vi "Create Hyperlink between 2 sheets.vi"(0 "Work Sheet":refnum<k7>, 1 "Sheet Name 2":string, 2 "Sheet Name 1":string, 3 "Link Cell 1":string, 4 "Link Cell 2":string, 5 "error in":errorcluster, 6 "File Path":path, 8 "Worksheets":refnum<k7>) -> (19 "error out":errorcluster)   [LabVIEW 2017]
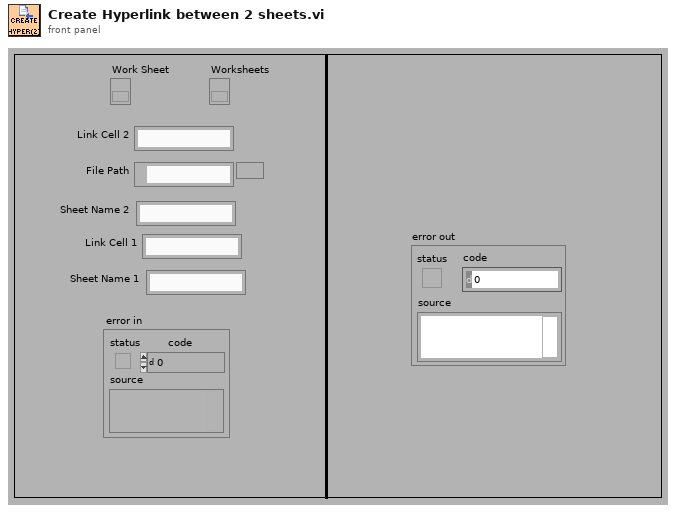
[diagram p1: front panel]
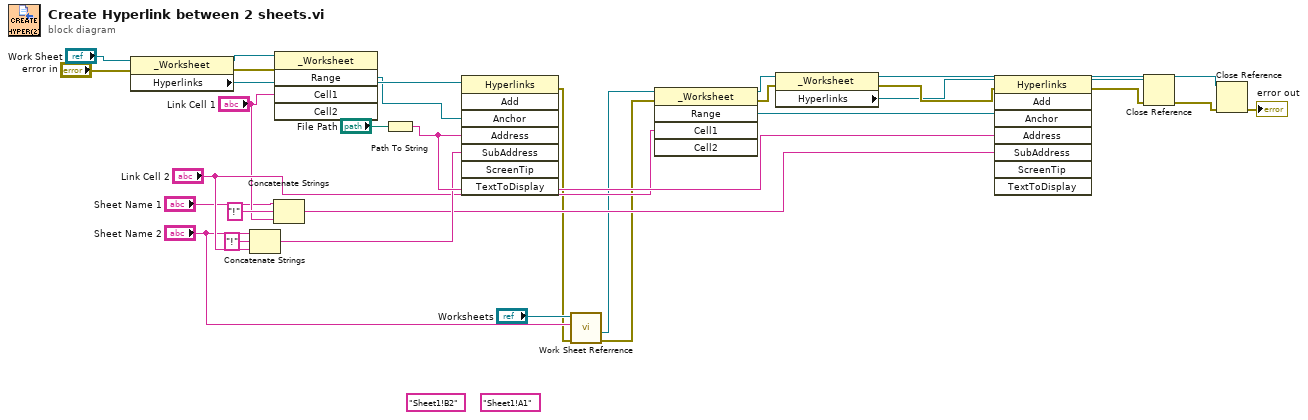
[diagram p0: block diagram]
diagram:
  (unwired) "Sheet1!A1"
  (unwired) "Sheet1!B2"
  n1 = property class="_Worksheet"(reference="Work Sheet", error in="error in") -> (reference out=w30:refnum<k7>, error out=w29:errorcluster, "Hyperlinks"=w28:refnum<k7>)
  n2 = Concatenate Strings("Sheet Name 2", "!" ("string"), "Link Cell 2") -> (w21:string)
  n3 = Concatenate Strings("Sheet Name 1", "!" ("string"), "Link Cell 1") -> (w17:string)
  n4 = invoke class="_Worksheet" method="Range"(reference=w30, error in=w29, "Cell1"="Link Cell 1") -> ("Range"=w27:refnum<k7>)  [unwired: 2 in, 4 out]
  n5 = Path To String(path="File Path") -> (string=w25:string)
  n6 = invoke class="Hyperlinks" method="Add"(reference=w28, "Anchor"=w27, "Address"=w25, "SubAddress"=w21) -> (error out=w11:errorcluster)  [unwired: 4 in, 7 out]
  n7 = call "Work Sheet Referrence.vi"("error in"=w11, "Sheet Name"="Sheet Name 2", "Worksheets 2"="Worksheets") -> ("error out"=w10:errorcluster, "Work Sheet"=w13:refnum<k7>)  [unwired: 7 out]
  n8 = invoke class="_Worksheet" method="Range"(reference=w13, error in=w10, "Cell1"="Link Cell 2") -> (reference out=w9:refnum<k7>, error out=w8:errorcluster, "Range"=w26:refnum<k7>)  [unwired: 2 in, 2 out]
  n9 = property class="_Worksheet"(reference=w9, error in=w8) -> (reference out=w3:refnum<k7>, error out=w7:errorcluster, "Hyperlinks"=w6:refnum<k7>)
  n10 = invoke class="Hyperlinks" method="Add"(reference=w6, error in=w7, "Anchor"=w26, "Address"=w25, "SubAddress"=w17) -> (reference out=w5:refnum<k7>, error out=w4:errorcluster)  [unwired: 3 in, 6 out]
  n11 = Close Reference(reference=w5, error in (no error)=w4) -> (error out=w2:errorcluster)
  n12 = Close Reference(reference=w3, error in (no error)=w2) -> (error out=→"error out":errorcluster)
